vi "Close Instrument.vi"(7 "Go Local (\"@LOC\")":bool, 8 "error in (no error)":errorcluster, 11 "Tektronix TDS 200 1000 2000 in":refnum<class "Tektronix TDS 200 1000 2000.lvclass">) -> (0 "error out":errorcluster, 3 "Tektronix TDS 200 1000 2000 out":refnum<class "Tektronix TDS 200 1000 2000.lvclass">)   [LabVIEW 2020, in "Tektronix TDS 200 1000 2000.lvclass"]
uses:
  Tektronix TDS 200 1000 2000.lvclass
  C:/Sandbox/Git_Sandbox/WiSpry Test Framework source code (LV20)/WiSpry Test Framework/Instruments/Instrument.lvclass
  Instrument.lvclass/Instrument.ctl
  Instrument.lvclass
  <instrlib>/Tektronix TDS 200 1000 2000 Series/Tektronix TDS 200 1000 2000 Series.lvlib
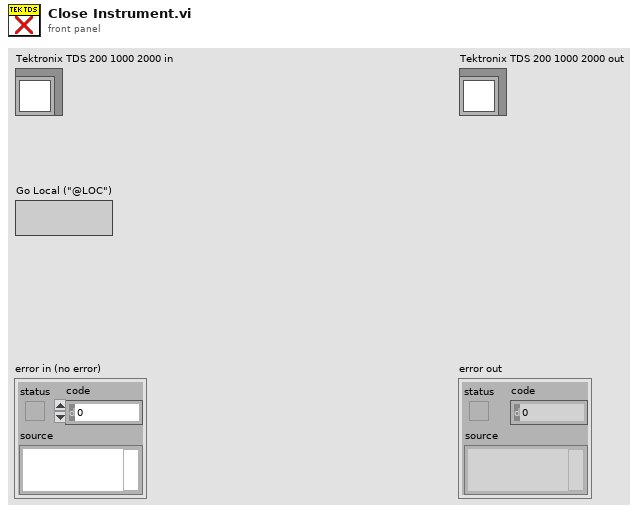
[diagram p1: front panel]
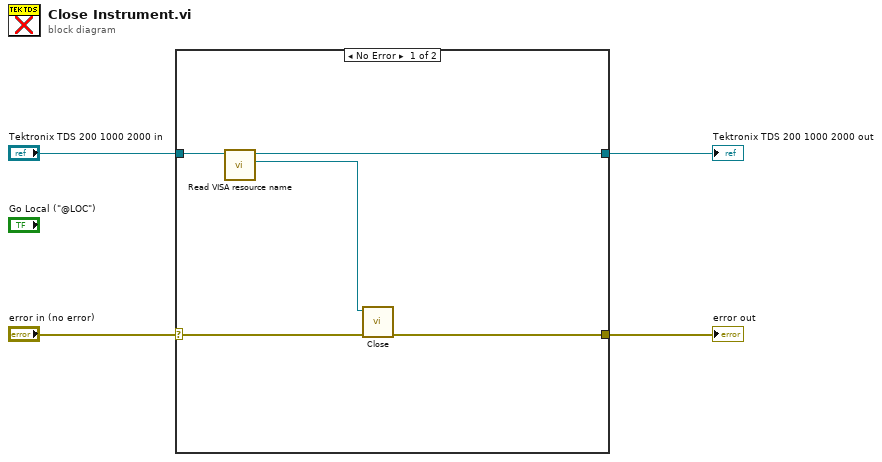
[diagram p0: block diagram]
diagram:
  n1 = case shown="No Error" "error in (no error)" {
    selector: "error in (no error)" -> [w7 w11]
    tunnel: [w6 w11] -> w1
    tunnel: [w8 w10] -> w2
    tunnel: "Tektronix TDS 200 1000 2000 in" -> [w9 w10]
    frame No Error {
      n2 = call "Read VISA resource name.vi"("Instrument in"=w9) -> ("VISA resource name"=w5:refnum<visa-resource-name>, "Instrument out"=w8:refnum<class "Tektronix TDS 200 1000 2000.lvclass">)  [unwired: 9 in]
      n3 = call <instrlib>:"Close.vi"("error in (no error)"=w7, "VISA resource name"=w5) -> ("error out"=w6:errorcluster)  [unwired: 9 in]
    }
    frame Error {
    }
  }
  "error out" <- w1
  "Tektronix TDS 200 1000 2000 out" <- w2
